vi "SetWaveforms.vi"(8 "error in (no error)":errorcluster, 10 "Waveforms":waveform(dbl)[](array[waveform]), 11 "FunctionBase in":refnum<class "FunctionBase.lvclass">) -> (0 "error out":errorcluster, 3 "FunctionBase out":refnum<class "FunctionBase.lvclass">)   [LabVIEW 2014, in "Functions.lvlib" / "FunctionBase.lvclass"]
uses:
  FunctionBase.lvclass
  FunctionBase.lvclass/FunctionBase.ctl
  Accessors/Write Waveforms.vi
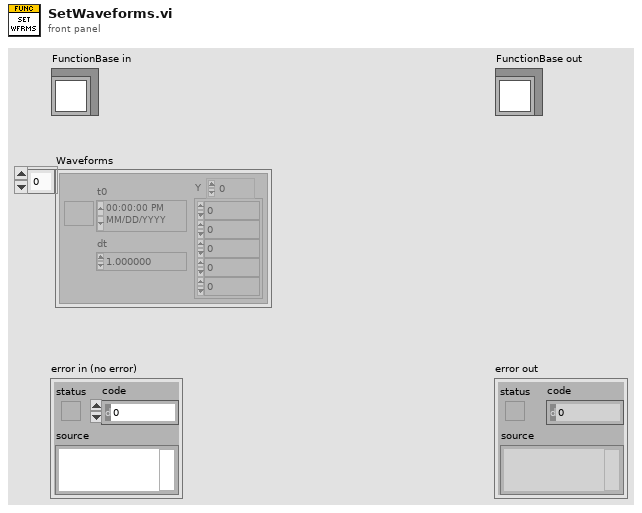
[diagram p1: front panel]
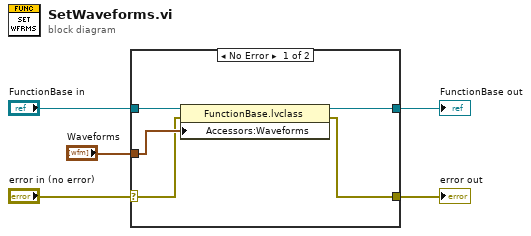
[diagram p0: block diagram]
diagram:
  n1 = case shown="No Error" "error in (no error)" {
    selector: "error in (no error)" -> [w7 w12]
    tunnel: [w6 w12] -> w4
    tunnel: [w9 w11] -> w2
    tunnel: "FunctionBase in" -> [w10 w11]
    tunnel: "Waveforms" -> [w8 _]
    frame No Error {
      n2 = property class="FunctionBase.lvclass"(reference=w10, error in=w7, "Accessors:Waveforms"=w8) -> (reference out=w9:refnum<class "FunctionBase.lvclass">, error out=w6:errorcluster)
    }
    frame Error {
    }
  }
  "error out" <- w4
  "FunctionBase out" <- w2
